vi "niDTS WLAN Rx Test UTIL Parameters to DUT Parameters.vi"(7 "Parameters":T1={"Standard"=enum."802.11 n HT", "DSSS Data Rate (Mbps)"=enum."1", "OFDM Data Rate (Mbps)"=enum."54", "MCS Index"=7, "N Spatial Streams"=1, "Chains"=[TRUE, FALSE, FALSE, FALSE], "Bandwidth (Hz)"=enum."20 MHz", "Channel"=1, "Power (dBm)"=0.0, "Guard Interval"=enum."SHORT", "FEC Coding"=enum."LDPC", "16 symbols"=TRUE, "Payload Length (bytes)"=1500, "Idle Interval (s)"=0.0001, "External Attenuation (dB)"=[0.0, 0.0, 0.0, 0.0], "RX Measurement Parameters"={"Number of Packets"=1000, "MacAddress"="FF:FF:FF:FF:FF:FF"}} {"Idle Interval (s)" format="%_3p"}) -> (8 "TV Parameters(DataType)":T9={"WLAN Type"=enum."b - 1 Mbps", "Bandwidth (Hz)"=enum."20 MHz", "Channel"=0, "Guard Interval"=enum."LONG", "FEC Coding"=enum."LDPC", "Power (dBm)"=0.0, "Payload Length (bytes)"=1500, "16 Symbols"=TRUE, "Chains"=[TRUE, FALSE, FALSE, FALSE]})   [LabVIEW 2015, in "niDTS WLAN.lvlib"]
uses:
  niDTS WLAN.lvlib
  Includes/niDTS WLAN DUT INC Parameters.ctl
  Includes/niDTS WLAN INC Type.ctl
  Includes/niDTS WLAN INC CH BW.ctl
  Includes/niDTS WLAN INC GI.ctl
  Includes/niDTS WLAN INC FEC Coding.ctl
  Includes/niDTS WLAN Rx Test INC Parameters.ctl
  Includes/niDTS WLAN INC Standard.ctl
  Includes/niDTS WLAN INC DSSS Data Rate.ctl
  Includes/niDTS WLAN INC OFDM Data Rate.ctl
  Includes/niDTS WLAN INC RX Measurement Parameters.ctl
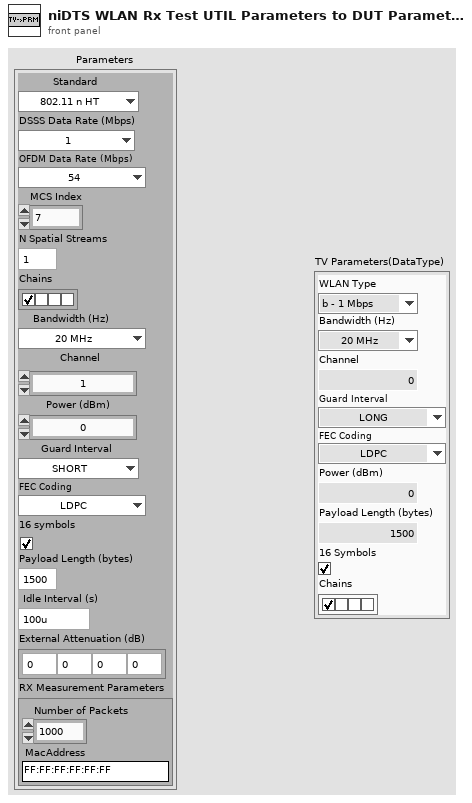
[diagram p1: front panel]
types:
  T1 = typedef "niDTS WLAN.lvlib/niDTS WLAN Rx Test INC Parameters.ctl" = cluster{"Standard":T2, "DSSS Data Rate (Mbps)":T3, "OFDM Data Rate (Mbps)":T4, "MCS Index":i32, "N Spatial Streams":i32, "Chains":bool[], "Bandwidth (Hz)":T5, "Channel":i32, "Power (dBm)":dbl, "Guard Interval":T6, "FEC Coding":T7, "16 symbols":bool, "Payload Length (bytes)":i32, "Idle Interval (s)":dbl, "External Attenuation (dB)":dbl[], "RX Measurement Parameters":T8}
  T2 = typedef "niDTS WLAN.lvlib/niDTS WLAN INC Standard.ctl" = enum16{"802.11 b DSSS", "802.11 a/g OFDM", "802.11 n HT", "802.11 ac VHT"}
  T3 = typedef "niDTS WLAN.lvlib/niDTS WLAN INC DSSS Data Rate.ctl" = enum16{"1", "2", "5.5", "11"}
  T4 = typedef "niDTS WLAN.lvlib/niDTS WLAN INC OFDM Data Rate.ctl" = enum16{"6", "9", "12", "18", "24", "36", "48", "54"}
  T5 = typedef "niDTS WLAN.lvlib/niDTS WLAN INC CH BW.ctl" = enum16{"20 MHz", "40 MHz", "80 MHz", "160 MHz"}
  T6 = typedef "niDTS WLAN.lvlib/niDTS WLAN INC GI.ctl" = enum16{"LONG", "SHORT"}
  T7 = typedef "niDTS WLAN.lvlib/niDTS WLAN INC FEC Coding.ctl" = enum16{"BCC", "LDPC"}
  T8 = typedef "niDTS WLAN.lvlib/niDTS WLAN INC RX Measurement Parameters.ctl" = cluster{"Number of Packets":i32, "MacAddress":string}
  T9 = typedef "niDTS WLAN.lvlib/niDTS WLAN DUT INC Parameters.ctl" = cluster{"WLAN Type":T10, "Bandwidth (Hz)":T5, "Channel":i32, "Guard Interval":T6, "FEC Coding":T7, "Power (dBm)":dbl, "Payload Length (bytes)":i32, "16 Symbols":bool, "Chains":bool[]}
  T10 = typedef "niDTS WLAN.lvlib/niDTS WLAN INC Type.ctl" = enum16{"b - 1 Mbps", "b - 2 Mbps", "b - 5.5 Mbps", "b - 11 Mbps", "ag - 6 Mbps", "ag - 9 Mbps", "ag - 12 Mbps", "ag - 18 Mbps", "ag - 24 Mbps", "ag - 36 Mbps", "ag - 48 Mbps", "ag - 54 Mbps", "n - MCS0", "n - MCS1", "n - MCS2", "n - MCS3", "n - MCS4", "n - MCS5", "n - MCS6", "n - MCS7", "n - MCS8", "n - MCS9", "n - MCS10", "n - MCS11", "n - MCS12", "n - MCS13", "n - MCS14", "n - MCS15", "n - MCS16", "n - MCS17", "n - MCS18", "n - MCS19", "n - MCS20", "n - MCS21", "n - MCS22", "n - MCS23", "n - MCS24", "n - MCS25", "n - MCS26", "n - MCS27", "n - MCS28", "n - MCS29", "n - MCS30", "n - MCS31", "ac - MCS0 -1", "ac - MCS1 -1", "ac - MCS2 -1", "ac - MCS3 -1", "ac - MCS4 -1", "ac - MCS5 -1", "ac - MCS6 -1", "ac - MCS7 -1", "ac - MCS8 -1", "ac - MCS9 -1", "ac - MCS0 -2", "ac - MCS1 -2", "ac - MCS2 -2", "ac - MCS3 -2", "ac - MCS4 -2", "ac - MCS5 -2", "ac - MCS6 -2", "ac - MCS7 -2", "ac - MCS8 -2", "ac - MCS9 -2", "ac - MCS0 -3", "ac - MCS1 -3", "ac - MCS2 -3", "ac - MCS3 -3", "ac - MCS4 -3", "ac - MCS5 -3", "ac - MCS6 -3", "ac - MCS7 -3", "ac - MCS8 -3", "ac - MCS9 -3", "ac - MCS0 -4", "ac - MCS1 -4", "ac - MCS2 -4", "ac - MCS3 -4", "ac - MCS4 -4", "ac - MCS5 -4", "ac - MCS6 -4", "ac - MCS7 -4", "ac - MCS8 -4", "ac - MCS9 -4"}
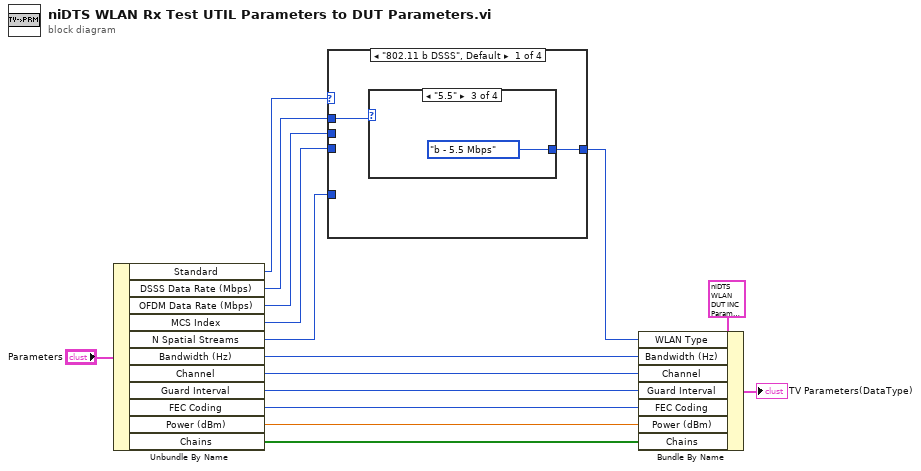
[diagram p0: block diagram]
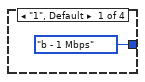
[diagram p2: hidden frame]
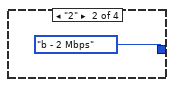
[diagram p3: hidden frame]
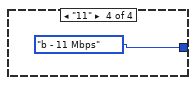
[diagram p4: hidden frame]
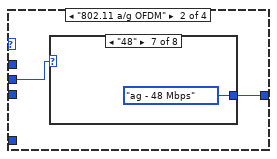
[diagram p5: hidden frame]
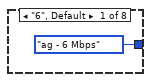
[diagram p6: hidden frame]
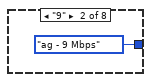
[diagram p7: hidden frame]
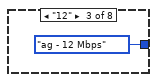
[diagram p8: hidden frame]
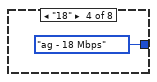
[diagram p9: hidden frame]
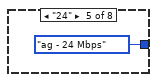
[diagram p10: hidden frame]
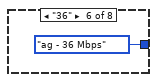
[diagram p11: hidden frame]
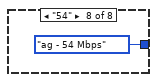
[diagram p12: hidden frame]
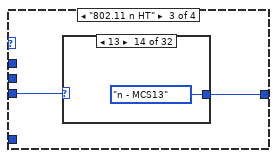
[diagram p13: hidden frame]
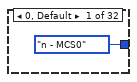
[diagram p14: hidden frame]
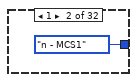
[diagram p15: hidden frame]
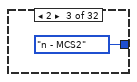
[diagram p16: hidden frame]
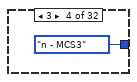
[diagram p17: hidden frame]
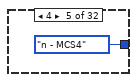
[diagram p18: hidden frame]
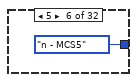
[diagram p19: hidden frame]
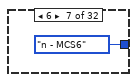
[diagram p20: hidden frame]
diagram:
  n1 = Unbundle By Name("Parameters") -> ("Standard"=w3:T2, "DSSS Data Rate (Mbps)"=w4:T3, "OFDM Data Rate (Mbps)"=w10:T4, "MCS Index"=w9:i32, "N Spatial Streams"=w5:i32, "Bandwidth (Hz)"=w8:T5, "Channel"=w7:i32, "Guard Interval"=w13:T6, "FEC Coding"=w1:T7, "Power (dBm)"=w6:dbl, "Chains"=w2:bool[])
  n2 = case shown="\"802.11 b DSSS\", Default" w3 {
    tunnel: w9 -> [_ _ w33 w72]
    tunnel: w10 -> [_ w23 _ _]
    tunnel: [w17 w22 w32 w68] -> w11
    tunnel: w5 -> [_ _ _ w67]
    tunnel: w4 -> [w16 _ _ _]
    frame "802.11 b DSSS", Default {
      n3 = case shown="\"5.5\"" w16 {
        tunnel: [niDTS_WLAN_INC_Type."b - 1 Mbps" ("WLAN Type 2") niDTS_WLAN_INC_Type."b - 2 Mbps" ("WLAN Type 2") niDTS_WLAN_INC_Type."b - 5.5 Mbps" ("WLAN Type 2") niDTS_WLAN_INC_Type."b - 11 Mbps" ("WLAN Type 2")] -> w17
        frame "1", Default {
        }
        frame "2" {
        }
        frame "5.5" {
        }
        frame "11" {
        }
      }
    }
    frame "802.11 a/g OFDM" {
      n4 = case shown="\"48\"" w23 {
        tunnel: [niDTS_WLAN_INC_Type."ag - 6 Mbps" ("WLAN Type 2") niDTS_WLAN_INC_Type."ag - 9 Mbps" ("WLAN Type 2") niDTS_WLAN_INC_Type."ag - 12 Mbps" ("WLAN Type 2") niDTS_WLAN_INC_Type."ag - 18 Mbps" ("WLAN Type 2") niDTS_WLAN_INC_Type."ag - 24 Mbps" ("WLAN Type 2") niDTS_WLAN_INC_Type."ag - 36 Mbps" ("WLAN Type 2") niDTS_WLAN_INC_Type."ag - 48 Mbps" ("WLAN Type 2") niDTS_WLAN_INC_Type."ag - 54 Mbps" ("WLAN Type 2")] -> w22
        frame "6", Default {
        }
        frame "9" {
        }
        frame "12" {
        }
        frame "18" {
        }
        frame "24" {
        }
        frame "36" {
        }
        frame "48" {
        }
        frame "54" {
        }
      }
    }
    frame "802.11 n HT" {
      n5 = case shown="13" w33 {
        tunnel: [niDTS_WLAN_INC_Type."n - MCS0" ("WLAN Type 2") niDTS_WLAN_INC_Type."n - MCS1" ("WLAN Type 2") niDTS_WLAN_INC_Type."n - MCS2" ("WLAN Type 2") niDTS_WLAN_INC_Type."n - MCS3" ("WLAN Type 2") niDTS_WLAN_INC_Type."n - MCS4" ("WLAN Type 2") niDTS_WLAN_INC_Type."n - MCS5" ("WLAN Type 2") niDTS_WLAN_INC_Type."n - MCS6" ("WLAN Type 2") niDTS_WLAN_INC_Type."n - MCS7" ("WLAN Type 2") niDTS_WLAN_INC_Type."n - MCS8" ("WLAN Type 2") niDTS_WLAN_INC_Type."n - MCS9" ("WLAN Type 2") niDTS_WLAN_INC_Type."n - MCS10" ("WLAN Type 2") niDTS_WLAN_INC_Type."n - MCS11" ("WLAN Type 2") niDTS_WLAN_INC_Type."n - MCS12" ("WLAN Type 2") niDTS_WLAN_INC_Type."n - MCS13" ("WLAN Type 2") niDTS_WLAN_INC_Type."n - MCS14" ("WLAN Type 2") niDTS_WLAN_INC_Type."n - MCS15" ("WLAN Type 2") niDTS_WLAN_INC_Type."n - MCS16" ("WLAN Type 2") niDTS_WLAN_INC_Type."n - MCS17" ("WLAN Type 2") niDTS_WLAN_INC_Type."n - MCS18" ("WLAN Type 2") niDTS_WLAN_INC_Type."n - MCS19" ("WLAN Type 2") niDTS_WLAN_INC_Type."n - MCS20" ("WLAN Type 2") niDTS_WLAN_INC_Type."n - MCS21" ("WLAN Type 2") niDTS_WLAN_INC_Type."n - MCS22" ("WLAN Type 2") niDTS_WLAN_INC_Type."n - MCS23" ("WLAN Type 2") niDTS_WLAN_INC_Type."n - MCS24" ("WLAN Type 2") niDTS_WLAN_INC_Type."n - MCS25" ("WLAN Type 2") niDTS_WLAN_INC_Type."n - MCS26" ("WLAN Type 2") niDTS_WLAN_INC_Type."n - MCS27" ("WLAN Type 2") niDTS_WLAN_INC_Type."n - MCS28" ("WLAN Type 2") niDTS_WLAN_INC_Type."n - MCS29" ("WLAN Type 2") niDTS_WLAN_INC_Type."n - MCS30" ("WLAN Type 2") niDTS_WLAN_INC_Type."n - MCS31" ("WLAN Type 2")] -> w32
        frame 0, Default {
        }
        frame 1 {
        }
        frame 2 {
        }
        frame 3 {
        }
        frame 4 {
        }
        frame 5 {
        }
        frame 6 {
        }
        frame 7 {
        }
        frame 8 {
        }
        frame 9 {
        }
        frame 10 {
        }
        frame 11 {
        }
        frame 12 {
        }
        frame 13 {
        }
        frame 14 {
        }
        frame 15 {
        }
        frame 16 {
        }
        frame 17 {
        }
        frame 18 {
        }
        frame 19 {
        }
        frame 20 {
        }
        frame 21 {
        }
        frame 22 {
        }
        frame 23 {
        }
        frame 24 {
        }
        frame 25 {
        }
        frame 26 {
        }
        frame 27 {
        }
        frame 28 {
        }
        frame 29 {
        }
        frame 30 {
        }
        frame 31 {
        }
      }
    }
    frame "802.11 ac VHT" {
      n6 = case shown="0, Default" w72 {
        tunnel: [niDTS_WLAN_INC_Type."ac - MCS0 -1" ("WLAN Type 2") niDTS_WLAN_INC_Type."ac - MCS1 -1" ("WLAN Type 2") niDTS_WLAN_INC_Type."ac - MCS2 -1" ("WLAN Type 2") niDTS_WLAN_INC_Type."ac - MCS3 -1" ("WLAN Type 2") niDTS_WLAN_INC_Type."ac - MCS4 -1" ("WLAN Type 2") niDTS_WLAN_INC_Type."ac - MCS5 -1" ("WLAN Type 2") niDTS_WLAN_INC_Type."ac - MCS6 -1" ("WLAN Type 2") niDTS_WLAN_INC_Type."ac - MCS7 -1" ("WLAN Type 2") niDTS_WLAN_INC_Type."ac - MCS8 -1" ("WLAN Type 2") niDTS_WLAN_INC_Type."ac - MCS9 -1" ("WLAN Type 2")] -> w71
        frame 0, Default {
        }
        frame 1 {
        }
        frame 2 {
        }
        frame 3 {
        }
        frame 4 {
        }
        frame 5 {
        }
        frame 6 {
        }
        frame 7 {
        }
        frame 8 {
        }
        frame 9 {
        }
      }
      n7 = Decrement(x=w67) -> (x-1=w66:i32)
      n8 = Multiply(x=w66, y=10) -> (x*y=w69:i32)
      n9 = Add(x=w71, y=w69) -> (x+y=w68:i32)
    }
  }
  n10 = Bundle By Name(cluster=T9 {"WLAN Type"=enum."b - 1 Mbps", "Bandwidth (Hz)"=enum."20 MHz", "Channel"=0, "Guard Interval"=enum."LONG", "FEC Coding"=enum."LDPC", "Power (dBm)"=0.0, "Payload Length (bytes)"=1500, "16 Symbols"=TRUE, "Chains"=[TRUE, FALSE, FALSE, FALSE]} ("TV Parameters(DataType) 2"), "WLAN Type"=w11, "Bandwidth (Hz)"=w8, "Channel"=w7, "Guard Interval"=w13, "FEC Coding"=w1, "Power (dBm)"=w6, "Chains"=w2) -> (→"TV Parameters(DataType)":T9)
